vi "add_NavSatFix_roslv.vi"(0 "msg in":string, 1 "frame_id":string, 2 "NavSatStatus":T2 {"service" items=["SERVICE_GPS"=1, "SERVICE_GLONASS"=2, "SERVICE_COMPASS"=4, "SERVICE_GALILEO"=8]; "status" items=["STATUS_NO_FIX"=-1, "STATUS_FIX"=0, "STATUS_SBAS_FIX"=1, "STATUS_GBAS_FIX"=2]}, 3 "Location":T1, 4 "position_covariance_type":u8(ring) items=["COVARIANCE_TYPE_UNKNOWN", "COVARIANCE_TYPE_APPROXIMATED", "COVARIANCE_TYPE_DIAGONAL_KNOWN", "COVARIANCE_TYPE_KNOWN"], 5 "position_covariance":dbl[](array[numeric])) -> (6 "msg out":string)   [LabVIEW 2014]
doc: "Creates a ROS sensor_msgs/NavSatFix message for use with a global positioning system."
uses:
  typedefs/msgs/NavSatStatus.ctl
  std_msgs/subs/float64Scalar_roslv.vi
  std_msgs/subs/u8Scalar_roslv.vi
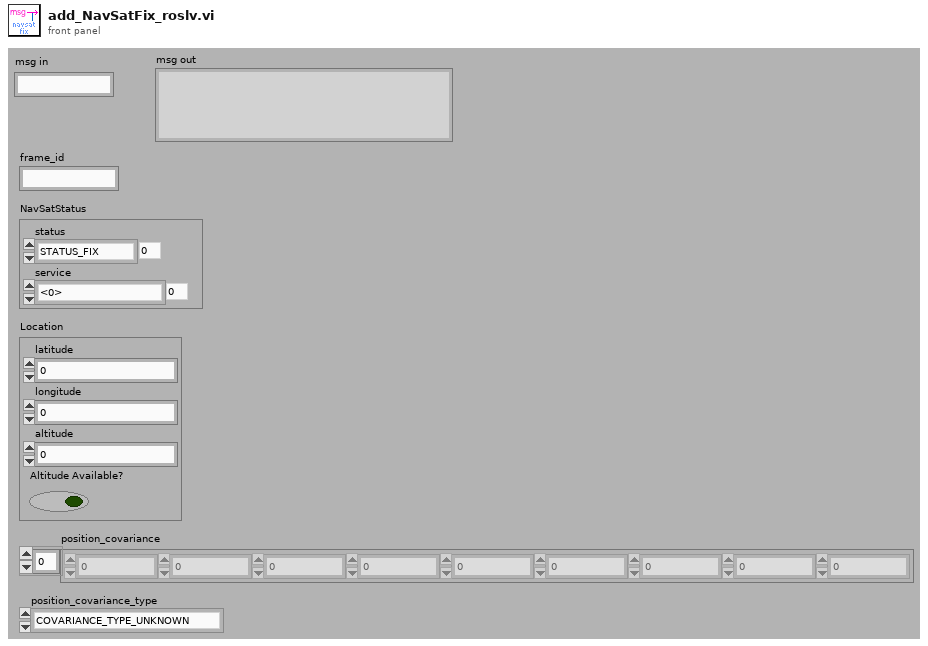
[diagram p1: front panel]
types:
  T1 = cluster{"latitude":dbl, "longitude":dbl, "altitude":dbl, "Altitude Available?":bool}
  T2 = typedef "NavSatStatus.ctl" = cluster{"status":i8, "service":u16}
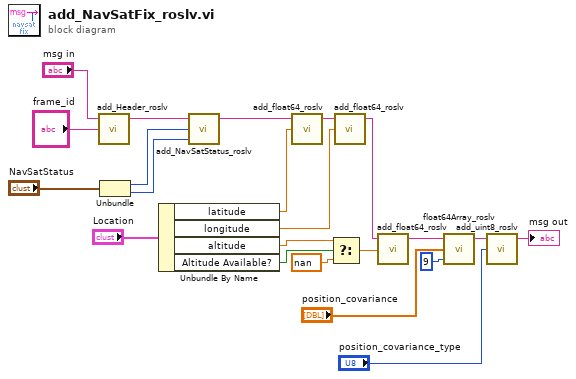
[diagram p0: block diagram]
diagram:
  n1 = call "add_Header_roslv.vi"("frame_id"="frame_id", "msg in"="msg in") -> ("msg out"=w20:string)  [unwired: 3 in]
  n2 = Unbundle("NavSatStatus") -> ("status"=w18:i8, "service"=w17:u16)
  n3 = Unbundle By Name("Location") -> ("latitude"=w13:dbl, "longitude"=w12:dbl, "altitude"=w9:dbl, "Altitude Available?"=w11:bool)
  n4 = call "add_NavSatStatus_roslv.vi"("service"=w17, "status"=w18, "msg in"=w20) -> ("msg out"=w7:string)  [unwired: 2 in]
  n5 = call-poly "add_float64_roslv.vi"("Numeric"=w13, "msg in"=w7) -> ("msg out"=w16:string)  [unwired: 3 in]
  n6 = Select(t=w9, s=w11, f=nan) -> (s? t:f=w8:dbl)
  n7 = call-poly "add_float64_roslv.vi"("Numeric"=w12, "msg in"=w16) -> ("msg out"=w15:string)  [unwired: 3 in]
  n8 = call-poly "add_float64_roslv.vi"("Numeric"=w8, "msg in"=w15) -> ("msg out"=w5:string)  [unwired: 3 in]
  n9 = call "float64Array_roslv.vi"("Array Length"=9, "Array"="position_covariance", "msg in"=w5) -> ("msg out"=w2:string)  [unwired: 2 in]
  n10 = call-poly "add_uint8_roslv.vi"("Numeric"="position_covariance_type", "msg in"=w2) -> ("msg out"=→"msg out":string)  [unwired: 3 in]
